vi "toml_load.vi"(8 "error in (no error)":errorcluster, 11 "path":path) -> (0 "error out":errorcluster, 3 "variant":variant)   [LabVIEW 2017]
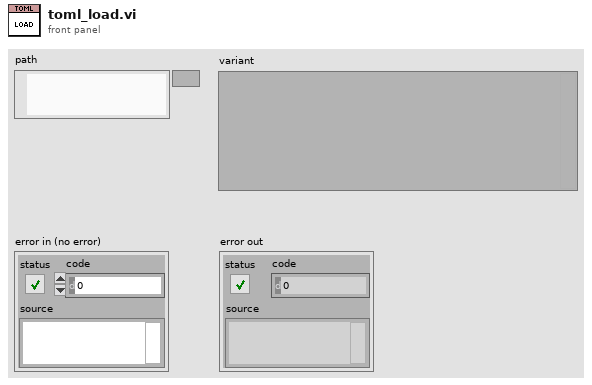
[diagram p1: front panel]
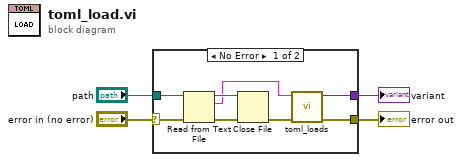
[diagram p0: block diagram]
diagram:
  n1 = case shown="No Error" "error in (no error)" {
    selector: "error in (no error)" -> [w12 w13]
    tunnel: "path" -> [w8 _]
    tunnel: [w6 w13] -> w2
    tunnel: [w5 _] -> w1
    frame No Error {
      n2 = Read from Text File(file (use dialog)=w8, error in=w12) -> (refnum out=w9:refnum<file>, text=w7:string, error out=w11:errorcluster)  [unwired: 2 in, 1 out]
      n3 = Close File(refnum=w9, error in=w11) -> (error out=w10:errorcluster)  [unwired: 1 out]
      n4 = call "toml_loads.vi"("error in (no error)"=w10, "toml"=w7) -> ("error out"=w6:errorcluster, "variant"=w5:variant)  [unwired: 8 in]
    }
    frame Error {
    }
  }
  "error out" <- w2
  "variant" <- w1
